vi "Stepper Move.vi"(0 "Instrument Address":refnum<visa-resource-name>, 1 "Motor Number":u32=1 min=1 max=255 step=1, 2 "Distance":dbl=1.0 min=-193273528.32 max=193273528.0 step=0.09 format="%.2f", 3 "error in (no error)":errorcluster, 4 "Mode":bool) -> (5 "error out":errorcluster)   [LabVIEW 2025]
doc: "Author: Scott Hannahs <sth@magnet.fsu.edu>\n\nThis software is licensed for use under the “MIT License\"\nCopyright (c) 2025 Scott Hannahs, sth@sth@magnet.sthnet.net\n\nPermission is hereby granted, free of charge, to any person obtaining a copy of this software and associated documentation files (the \"Software\"), to deal in the Software without restriction, including without limitation the rights to use, copy, modify, merge, publish, distribute, sublicense, and/or sell copies of the Software, and to permit persons to whom the Software is furnished to do so, subject to the following conditions: The above copyright notice and this permission notice shall be included in all copies or substantial portions of the Software.\n\nTHE SOFTWARE IS PROVIDED \"AS IS\", WITHOUT WARRANTY OF ANY KIND, EXPRESS OR IMPLIED, INCLUDING BUT NOT LIMITED TO THE WARRANTIES OF MERCHANTABILITY, FITNESS FOR A PARTICULAR PURPOSE AND NONINFRINGEMENT. IN NO EVENT SHALL THE AUTHORS OR COPYRIGHT HOLDERS BE LIABLE FOR ANY CLAIM, DAMAGES OR OTHER LIABILITY, WHETHER IN AN ACTION OF CONTRACT, TORT OR OTHERWISE, ARISING FROM, OUT OF OR IN CONNECTION WITH THE SOFTWARE OR THE USE OR OTHER DEALINGS IN THE SOFTWARE."
uses:
  Parker Stepper Global.vi
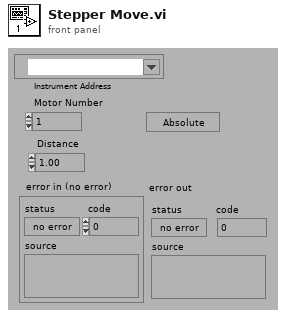
[diagram p1: front panel]
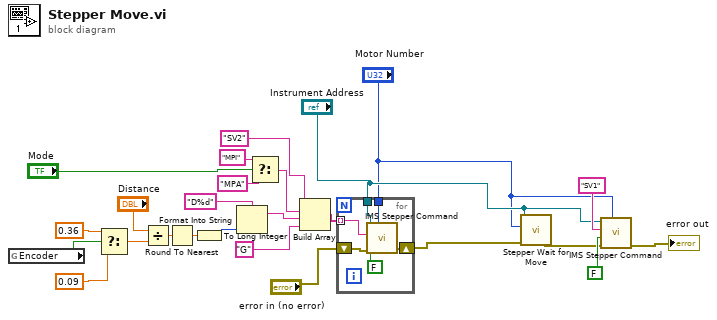
[diagram p0: block diagram]
diagram:
  n1 = global read "Parker Stepper Global.vi" "Encoder"() -> (w12:bool)
  n2 = Select(t=0.36 ("y"), s=w12, f=0.09 ("y")) -> (s? t:f=w13:dbl)
  n3 = Divide(x="Distance", y=w13) -> (x/y=w18:dbl)
  n4 = Round To Nearest(number=w18) -> (nearest integer value=w11:dbl)
  n5 = To Long Integer(number=w11) -> (32bit integer=w16:i32)
  n6 = Format Into String(format string="D%d", w16) -> (resulting string=w17:string)  [unwired: 2 in, 1 out]
  n7 = Select(t="MPI", s="Mode", f="MPA") -> (s? t:f=w20:string)
  n8 = Build Array("SV2", w20, w17, "G") -> (w19:string[])
  n9 = for {
    shift-right: [w31] -> w3
    shift-left: "error in (no error)" -> [w30]
    tunnel: w19 -> [w28] mode=indexing
    tunnel: "Instrument Address" -> [w27]
    tunnel: "Motor Number" -> [w26]
    n10 = call "IMS Stepper Command.vi"("Motor Number"=w26, "error in (no error)"=w30, "Mode"=FALSE, "Command"=w28, "Instrument Address"=w27) -> ("error out"=w31:errorcluster)  [unwired: 1 in, 3 out]
  }
  n11 = call "Stepper Wait for Move.vi"("Instrument Address"="Instrument Address", "Motor Number"="Motor Number", "error in (no error)"=w3) -> ("error out"=w4:errorcluster)  [unwired: 2 in]
  n12 = call "IMS Stepper Command.vi"("Motor Number"="Motor Number", "error in (no error)"=w4, "Mode"=FALSE, "Command"="SV1", "Instrument Address"="Instrument Address") -> ("error out"=→"error out":errorcluster)  [unwired: 1 in, 3 out]
